vi "Version Patch.vi"(6 "LabPack Shared Library":path=path "", 8 "Error In":errorcluster) -> (0 "Error Out":errorcluster, 3 "Version Patch":u32)   [LabVIEW 2019, in "LabPack.lvlib"]
doc: "Gets the Patch version number of the LabPack shared library. The LabPack shared library maintains a semantic versioning number with a Major, Minor, and Patch component. A difference in the Major number indicates backwards compatible breaking changes. A difference in the Minor number indicates new features and fixes that do not break backwards compatibility. A difference in the Patch number indicates a fix that does not break backwards compatibility and does not add any new features."
uses:
  LabPack.lvlib
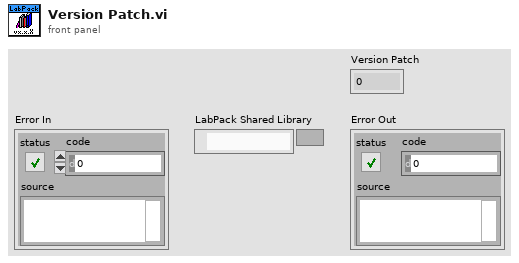
[diagram p1: front panel]
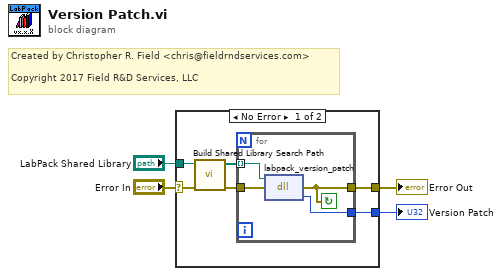
[diagram p0: block diagram]
diagram:
  # "Created by Christopher R. Field <chris@fieldrndservices.com>\n\nCopyright 2017 Field R&D Services, LLC"
  n1 = case shown="No Error" "Error In" {
    selector: "Error In" -> [w8 w15]
    tunnel: [w10 w15] -> w4
    tunnel: [w9 _] -> w2
    tunnel: "LabPack Shared Library" -> [w5 _]
    frame No Error {
      n2 = call "Build Shared Library Search Path.vi"("Error In"=w8, "LabPack Shared Library"=w5) -> ("Error Out"=w7:errorcluster, "Search Path"=w6:path[])  [unwired: 8 in]
      n3 = for {
        tunnel: [w14] -> w9
        tunnel: w6 -> [w12] mode=indexing
        tunnel: w7 -> [w13]
        tunnel: [w11] -> w10
        stop <- w11 continue-if-true
        n4 = dll-call lib="D:/Users/cfield/Code/MessagePack/LabPack/LabVIEW/trunk/src/LabPack/Private/labpack-x64.dll" fn="labpack_version_patch"(path in=w12, error in=w13) -> (error out=w11:errorcluster, "return type"=w14:u32)  [unwired: 1 in, 1 out]
      }
    }
    frame Error {
    }
  }
  "Error Out" <- w4
  "Version Patch" <- w2
